vi "ReadOptical.vi"(8 "OpticalOff":u32, 9 "OpticalHead":T1, 11 "RefIn":refnum<file>) -> (2 "PicOut":picture, 3 "RGBarray":u32[][](array[numeric]), 4 "RefOut":refnum<file>)   [LabVIEW 2012]
uses:
  ImageHeaderType.ctl
  <vilib>/picture/picture.llb/Draw True-Color Pixmap.vi
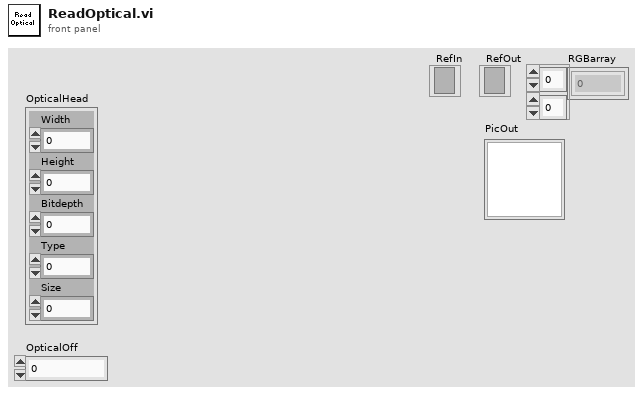
[diagram p1: front panel]
types:
  T1 = typedef "ImageHeaderType.ctl" = cluster{"Width":u32, "Height":u32, "Bitdepth":u32, "Type":u32, "Size":u32}
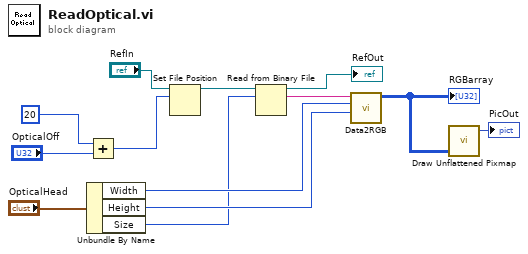
[diagram p0: block diagram]
diagram:
  n1 = Unbundle By Name("OpticalHead") -> ("Width"=w9:u32, "Height"=w8:u32, "Size"=w3:u32)
  n2 = Add(x=u32 20, y="OpticalOff") -> (x+y=w4:u32)
  n3 = Set File Position(offset (in bytes) (0)=w4, refnum="RefIn") -> (refnum out=w13:refnum<file>)  [unwired: 2 in, 1 out]
  n4 = Read from Binary File(10:w3, 11:w13) -> (2:w12:string, 3:→"RefOut":refnum<file>)  [unwired: 4 in, 2 out]
  n5 = call "Data2RGB.vi"("SizeY"=w8, "SizeX"=w9, "Data"=w12) -> ("RGBarray"=w2:u32[][])  [unwired: 8 in]
  "RGBarray" <- w2
  n6 = call-poly <vilib>:"Draw Unflattened Pixmap.vi"("data (RGB format)"=w2) -> ("new picture"=→"PicOut":picture)  [unwired: 8 in]
